vi "Configure High Speed USB Compliance Tests.vi"(6 "Internal Hubs (0)":i32, 7 "Connection Type (0: Singleended)":u16(ring) items=["Singleended", "Differential"], 8 "error in (no error)":errorcluster, 9 "Test Type (0: Nearend)":u16(ring) items=["Nearend", "Farend"], 10 "Differential Probe Channel (1: Ch 1)":u16(ring)=1 items=["Ch 1"=1, "Ch 2"=2, "Ch 3"=3, "Ch 4"=4], 11 "VISA resource name":refnum<visa-resource-name>) -> (0 "error out":errorcluster, 3 "VISA resource name out":refnum<visa-resource-name>)   [LabVIEW 2015, in "Agilent 2000 3000 X-Series.lvlib"]
doc: "Configures parameters for high speed USB tests.\n\nNote:\nThis VI is not supported by EDUX1052A/G, DSOX1202A/G, DSOX1204A/G models"
uses:
  Agilent 2000 3000 X-Series.lvlib
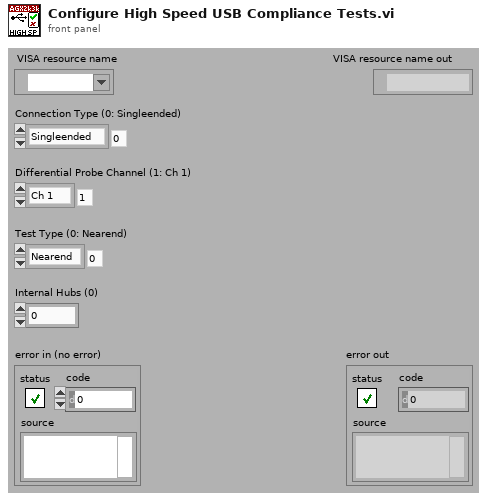
[diagram p1: front panel]
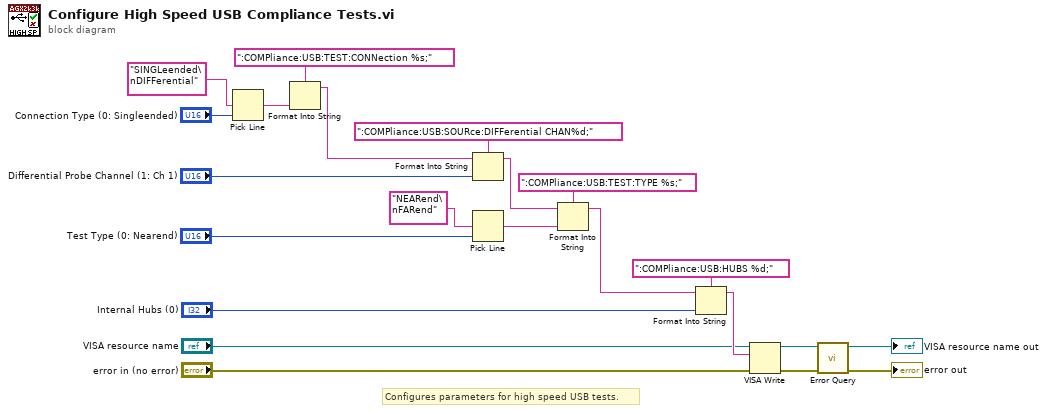
[diagram p0: block diagram]
diagram:
  # "Configures parameters for high speed USB tests."
  n1 = Pick Line(multi-line string="SINGLeended\nDIFFerential", line index="Connection Type (0: Singleended)") -> (output string=w19:string)  [unwired: 1 in]
  n2 = Format Into String(format string=":COMPliance:USB:TEST:CONNection %s;", w19) -> (resulting string=w2:string)  [unwired: 2 in, 1 out]
  n3 = Format Into String(format string=":COMPliance:USB:SOURce:DIFFerential CHAN%d;", initial string=w2, "Differential Probe Channel (1: Ch 1)") -> (resulting string=w1:string)  [unwired: 1 in, 1 out]
  n4 = Pick Line(multi-line string="NEARend\nFARend", line index="Test Type (0: Nearend)") -> (output string=w13:string)  [unwired: 1 in]
  n5 = Format Into String(format string=":COMPliance:USB:TEST:TYPE %s;", initial string=w1, w13) -> (resulting string=w10:string)  [unwired: 1 in, 1 out]
  n6 = Format Into String(format string=":COMPliance:USB:HUBS %d;", initial string=w10, "Internal Hubs (0)") -> (resulting string=w9:string)  [unwired: 1 in, 1 out]
  n7 = VISA Write(VISA resource name="VISA resource name", write buffer=w9, error in (no error)="error in (no error)") -> (VISA resource name out=w8:refnum<visa-resource-name>, error out=w7:errorcluster)  [unwired: 1 out]
  n8 = call "Error Query.vi"("error in (no error)"=w7, "VISA resource name"=w8) -> ("error out"=→"error out":errorcluster, "VISA resource name out"=→"VISA resource name out":refnum<visa-resource-name>)  [unwired: 6 in, 2 out]
